vi "Logic_Get_List_of_Devices.vi"(4 "error in (no error)":errorcluster, 6 "Include Simulated Devices?":bool, 7 "Session Ref In":T2) -> (0 "error out":errorcluster, 2 "Detected Devices":T1(array[cluster]), 3 "Session Ref Out":T2)   [LabVIEW 2023]
doc: "Open connection to the Saleae Logic2 software."
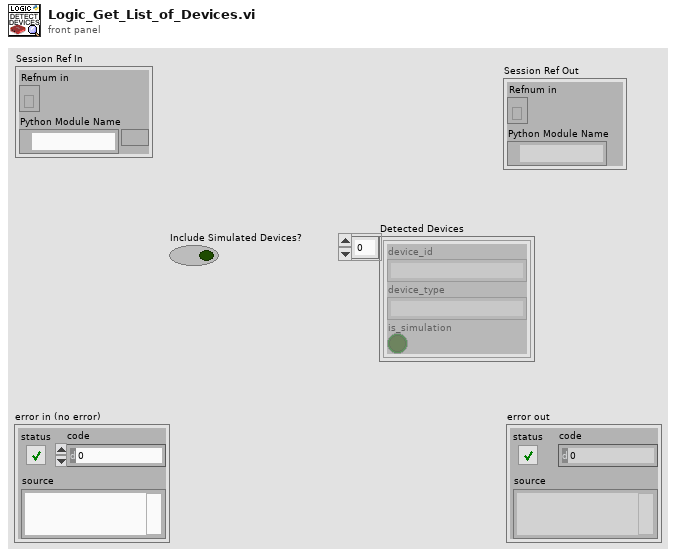
[diagram p1: front panel]
types:
  T1 = cluster{"device_id":string, "device_type":string, "is_simulation":bool}[]
  T2 = cluster{"Refnum in":refnum<k35>, "Python Module Name":path}
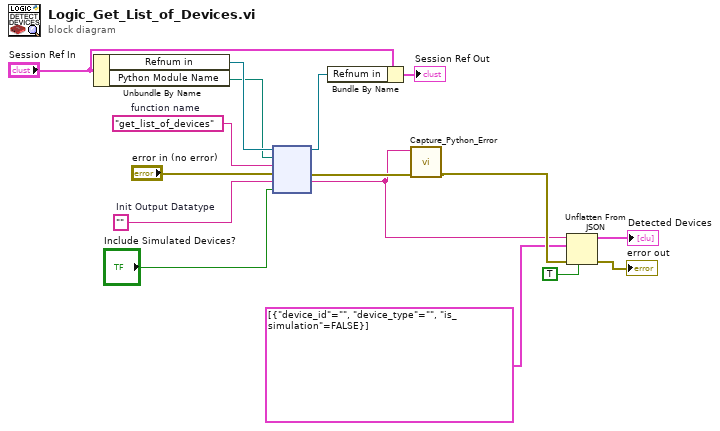
[diagram p0: block diagram]
diagram:
  w15 = "get_list_of_devices"  # function name
  w14 = ""  # Init Output Datatype
  n1 = Unbundle By Name("Session Ref In") -> ("Refnum in"=w10:refnum<k35>, "Python Module Name"=w9:path)
  n2 = node(w10, w9, w15, "error in (no error)", w14, "Include Simulated Devices?") -> (w8:refnum<k35>, w13:errorcluster, w2:string)  [unwired: 1 in, 2 out]
  n3 = Bundle By Name(cluster="Session Ref In", "Refnum in"=w8) -> (→"Session Ref Out":T2)
  n4 = call "Capture_Python_Error.vi"("error in (no error)"=w13, "Error Message (start with ERROR)"=w2) -> ("error out"=w7:errorcluster)  [unwired: 9 in]
  n5 = Unflatten From JSON(JSON string=w2, type and defaults=T1 [{"device_id"="", "device_type"="", "is_simulation"=FALSE}], default null elements? (F)=TRUE, error in (no error)=w7) -> (value=→"Detected Devices":T1, error out=→"error out":errorcluster)  [unwired: 3 in]
